vi "HelloWorld_LV18Nodes.vi"() -> ()   [LabVIEW 2018]
uses:
  <vilib>/ptbypt/NI_PtbyPt.lvlib
panel:
  out "Mean Execution Time (s)":dbl
  out "Execution Time":dbl(graph)
  out "Output":string
  out "Error Out":errorcluster
  in  "Name":string="World"
  in  "stop":bool
  # "This VI Demonstrates using the LabVIEW 2018 Python Nodes and benchmarks its execution time for comparison with other methods of communicating with Python in LabVIEW.\n\n1. Enter your name in the Name input to be personally greeted\n2. Run the VI"
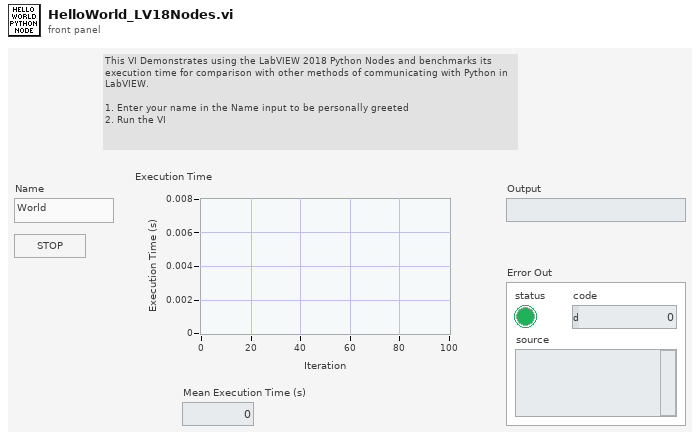
[diagram p1: front panel]
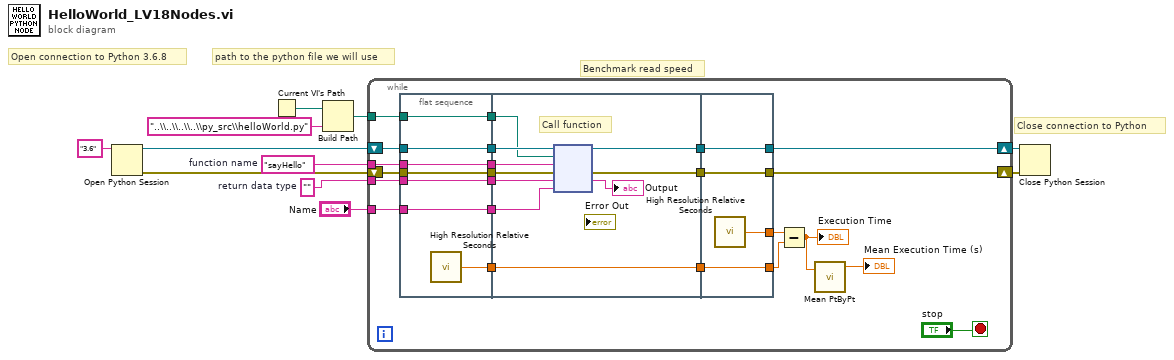
[diagram p0: block diagram]
diagram:
  w5 = ""  # return data type
  w6 = "sayHello"  # function name
  # "Close connection to Python"
  # "Benchmark read speed"
  # "Open connection to Python 3.6.8"
  # "path to the python file we will use"
  n1 = Open Python Session(python version="3.6" ("Python version")) -> (session out=w11:refnum<k35>, error out=w10:errorcluster)  [unwired: 2 in]
  n2 = Current VI's Path() -> (path=w3:path)
  n3 = Build Path(base path=w3, name or relative path="..\\..\\..\\..\\py_src\\helloWorld.py") -> (appended path=w1:path)
  n4 = while {
    tunnel: w1 -> [w30]
    tunnel: w6 -> [w29]
    tunnel: w5 -> [w28]
    tunnel: "Name" -> [w27]
    shift-right: [w32] -> w9
    shift-left: w11 -> [w34]
    shift-right: [w31] -> w8
    shift-left: w10 -> [w33]
    stop <- "stop" stop-if-true
    n5 = flat-sequence {
      tunnel: w27 -> [w36]
      tunnel: w28 -> [w37]
      tunnel: w29 -> [w38]
      tunnel: w30 -> [w39]
      tunnel: w33 -> [w40]
      tunnel: w34 -> [w41]
      tunnel: [w41] -> w23
      tunnel: [w40] -> w22
      tunnel: [w39] -> w21
      tunnel: [w38] -> w20
      tunnel: [w37] -> w19
      tunnel: [w36] -> w18
      tunnel: [w35] -> w16
      tunnel: [w49] -> w25
      tunnel: [w48] -> w24
      tunnel: w23 -> [w51]
      tunnel: w22 -> [w50]
      tunnel: w21 -> [w47]
      tunnel: w20 -> [w46]
      tunnel: w19 -> [w45]
      tunnel: w18 -> [w44]
      tunnel: [w43] -> w17
      tunnel: w16 -> [w43]
      tunnel: [w54] -> w31
      tunnel: [w55] -> w32
      tunnel: w25 -> [w55]
      tunnel: w24 -> [w54]
      tunnel: [w53] -> w15
      tunnel: [w52] -> w14
      tunnel: w17 -> [w52]
      frame #0 {
        n6 = call <vilib>:"High Resolution Relative Seconds.vi"() -> ("relative seconds"=w35:dbl)
      }
      frame #1 {
        # "Call function"
        n7 = node(w51, w47, w46, w50, w45, w44) -> (w49:refnum<k35>, w48:errorcluster, →"Output":string)  [unwired: 1 in, 2 out]
      }
      frame #2 {
        n8 = call <vilib>:"High Resolution Relative Seconds.vi"() -> ("relative seconds"=w53:dbl)
      }
    }
    n9 = Subtract(x=w15, y=w14) -> (x-y=w13:dbl)
    "Execution Time" <- w13
    n10 = call <vilib>:"Mean PtByPt.vi"("x"=w13) -> ("mean"=→"Mean Execution Time (s)":dbl)  [unwired: 3 in, 1 out]
  }
  n11 = Close Python Session(session in=w9, error in=w8) -> ()  [unwired: 1 out]
